vi "saveLogEntry.vi"(8 "error in (no error)":errorcluster, 11 "Logger in":refnum<class "TestDataLog.lvclass">) -> (0 "error out":errorcluster, 3 "Logger out":refnum<class "TestDataLog.lvclass">)   [LabVIEW 2013, in "TestDataLog.lvclass"]
uses:
  TestDataLog.lvclass
  TestDataLog.lvclass/TestDataLog.ctl
  <userlib>/Common/Log/Log/Log.lvclass/Log.ctl
  <userlib>/Common/Log/Log/Log.lvclass
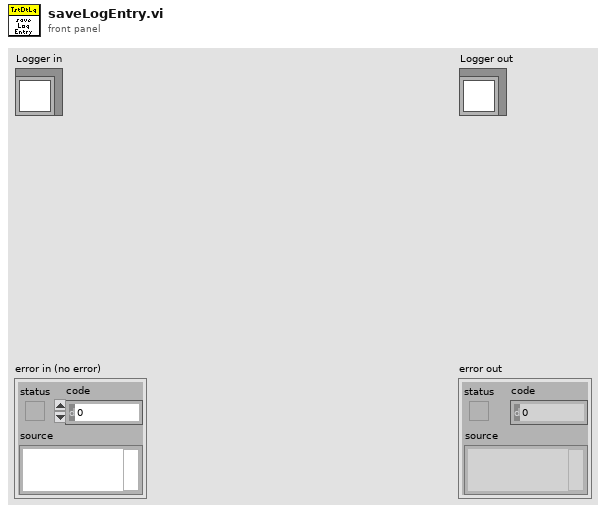
[diagram p1: front panel]
types:
  T1 = typedef "AITDTTypedefs.lvlib/InputData.ctl" = cluster{"Temperature Measured":dbl[unit], "ADCs":T2}
  T2 = typedef "ILCCommon.lvlib/ILCTypedefs.lvlib/ADCs.ctl" = cluster{"Ch0":i32, "Ch1":i32, "Ch2":i32, "Ch3":i32, "Ch4":i32}
  T3 = typedef "AITDTTypedefs.lvlib/StateSelector.ctl" = enum16{"AwaitingSetpointAcknowledgmentState", "EndingCycleState", "FaultState", "OffState", "PausingState", "RequestingNewSetpointState", "SamplingState", "SettlingState", "SoakingState", "StabilizingState", "StandbyState", "StoppedState", "TransitioningTemperatureState"}
  T4 = typedef "AITDTTypedefs.lvlib/TestStatus.ctl" = cluster{"activeCycle":u32, "activeProfileStep":u32, "demandedCycles":u32, "demandedProfileSteps":u32, "temperatureSetpoint":dbl[unit], "pgaGainCoefficient":u16}
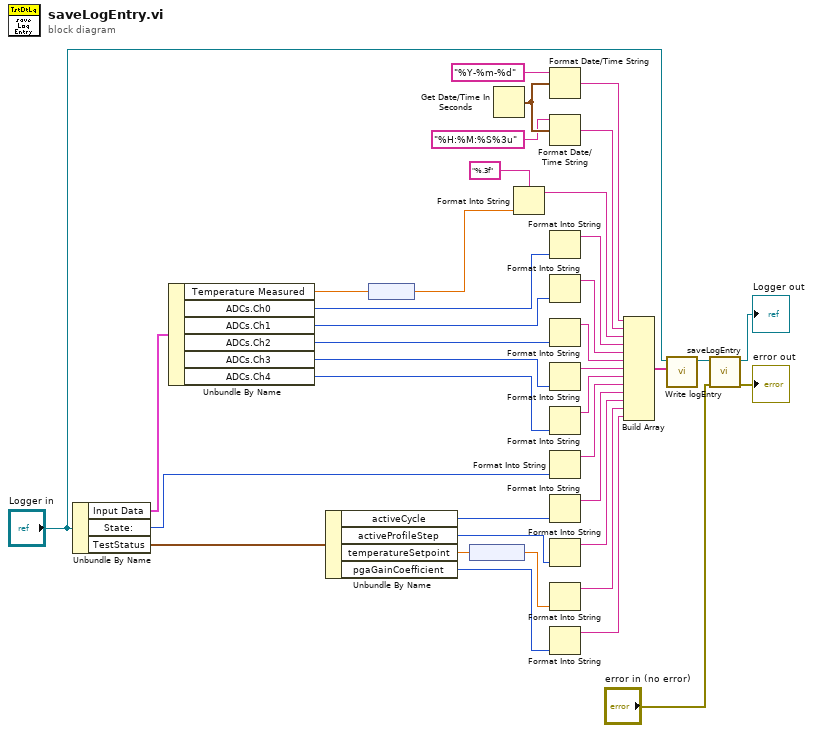
[diagram p0: block diagram]
diagram:
  n1 = Unbundle By Name("Logger in") -> ("Input Data"=w38:T1, "State:"=w36:T3, "TestStatus"=w33:T4)
  n2 = Unbundle By Name(w38) -> ("Temperature Measured"=w16:dbl[unit], "ADCs.Ch0"=w15:i32, "ADCs.Ch1"=w13:i32, "ADCs.Ch2"=w11:i32, "ADCs.Ch3"=w9:i32, "ADCs.Ch4"=w7:i32)
  n3 = Unbundle By Name(w33) -> ("activeCycle"=w32:u32, "activeProfileStep"=w31:u32, "temperatureSetpoint"=w5:dbl[unit], "pgaGainCoefficient"=w2:u16)
  n4 = node(w16) -> (w17:dbl)
  n5 = node(w5) -> (w4:dbl)
  n6 = Get Date/Time In Seconds() -> (seconds since 1Jan1904=w27:timestamp)
  n7 = Format Into String(format string="%.3f", w17) -> (resulting string=w37:string)  [unwired: 2 in, 1 out]
  n8 = Format Date/Time String(time format string (%c)="%Y-%m-%d" ("format string"), seconds (now)=w27) -> (date/time string=w24:string)  [unwired: 1 in]
  n9 = Format Date/Time String(time format string (%c)="%H:%M:%S%3u", seconds (now)=w27) -> (date/time string=w25:string)  [unwired: 1 in]
  n10 = Format Into String(w15) -> (resulting string=w14:string)  [unwired: 3 in, 1 out]
  n11 = Format Into String(w13) -> (resulting string=w12:string)  [unwired: 3 in, 1 out]
  n12 = Format Into String(w11) -> (resulting string=w10:string)  [unwired: 3 in, 1 out]
  n13 = Format Into String(w9) -> (resulting string=w8:string)  [unwired: 3 in, 1 out]
  n14 = Format Into String(w7) -> (resulting string=w6:string)  [unwired: 3 in, 1 out]
  n15 = Format Into String(w36) -> (resulting string=w35:string)  [unwired: 3 in, 1 out]
  n16 = Format Into String(w32) -> (resulting string=w30:string)  [unwired: 3 in, 1 out]
  n17 = Format Into String(w31) -> (resulting string=w29:string)  [unwired: 3 in, 1 out]
  n18 = Format Into String(w4) -> (resulting string=w3:string)  [unwired: 3 in, 1 out]
  n19 = Format Into String(w2) -> (resulting string=w1:string)  [unwired: 3 in, 1 out]
  n20 = Build Array(w24, w25, w37, w14, w12, w10, w8, w6, w35, w30, w29, w3, w1) -> (w21:string[])
  n21 = call <userlib>:"Write logEntry.vi"("logEntry"=w21, "Logger in"="Logger in") -> ("Logger out"=w22:refnum<class "TestDataLog.lvclass">)  [unwired: 9 in]
  n22 = call-parent "saveLogEntry.vi"("error in (no error)"="error in (no error)", "Logger in"=w22) -> ("error out"=→"error out":errorcluster, "Logger out"=→"Logger out":refnum<class "TestDataLog.lvclass">)  [unwired: 8 in]
